vi "rethinkdb_tcp_read.vi"(6 "timeout ms (10000)":i32=10000, 8 "error in (no error)":errorcluster, 11 "rethinkdb in":refnum<k5>) -> (0 "error out":errorcluster, 2 "data out":string, 3 "rethinkdb out":refnum<k5>)   [LabVIEW 2017]
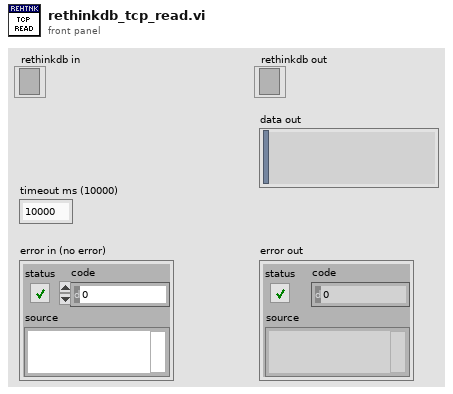
[diagram p1: front panel]
types:
  T1 = enum16{"Standard", "Buffered", "CRLF", "Immediate"}
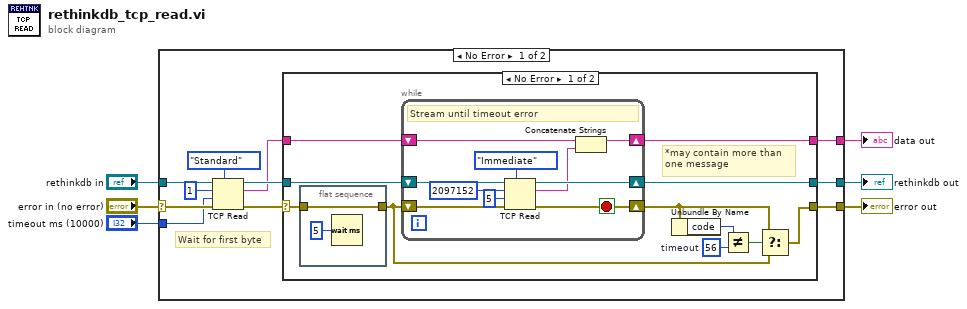
[diagram p0: block diagram]
diagram:
  n1 = case shown="No Error" "error in (no error)" {
    selector: "error in (no error)" -> [w16 w45]
    tunnel: "rethinkdb in" -> [w17 w44]
    tunnel: "timeout ms (10000)" -> [w15 _]
    tunnel: [w12 w45] -> w3
    tunnel: [w10 w44] -> w2
    tunnel: [w7 _] -> w1
    frame No Error {
      # "Wait for first byte"
      n2 = TCP Read(connection ID=w17, bytes to read=1, error in (no error)=w16, 7:T1."Standard" ("mode (standard)"), 9:w15) -> (connection ID out=w9:refnum<k5>, data out=w8:string, error out=w11:errorcluster)
      n3 = case shown="No Error" w11 {
        selector: w11 -> [w28 w43]
        tunnel: [w19 w43] -> w12
        tunnel: [w26 w42] -> w10
        tunnel: w9 -> [w27 w42]
        tunnel: w8 -> [w25 w41]
        tunnel: [w24 w41] -> w7
        frame No Error {
          w22 = 56  # timeout
          # "*may contain more than\none message"
          n4 = flat-sequence {
            tunnel: [w39] -> w18
            tunnel: w28 -> [w39]
            frame #0 {
              n5 = Wait (ms)(milliseconds to wait=u32 5) -> ()  [unwired: 1 out]
            }
          }
          n6 = while {
            shift-right: [w30] -> w20
            shift-left: w18 -> [w38]
            shift-right: [w36] -> w26
            shift-left: w27 -> [w37]
            shift-right: [w29] -> w24
            shift-left: w25 -> [w32]
            stop <- w30 stop-if-true
            # "Stream until timeout error"
            n7 = TCP Read(connection ID=w37, bytes to read=2097152, error in (no error)=w38, 7:T1."Immediate" ("mode (standard)"), 9:5 ("timeout ms (25000)")) -> (connection ID out=w36:refnum<k5>, data out=w31:string, error out=w30:errorcluster)
            n8 = Concatenate Strings(w32, w31) -> (w29:string)
          }
          n9 = Unbundle By Name(w20) -> ("code"=w23:i32)
          n10 = Not Equal?(x=w23, y=w22) -> (x != y?=w21:bool)
          n11 = Select(t=w20, s=w21, f=w18) -> (s? t:f=w19:errorcluster)
        }
        frame Error {
        }
      }
    }
    frame Error {
    }
  }
  "error out" <- w3
  "rethinkdb out" <- w2
  "data out" <- w1
